vi "CloseUDP Connection.vi"(5 "UDP Network Connection Refnum":refnum<k16>) -> ()   [LabVIEW 2013]
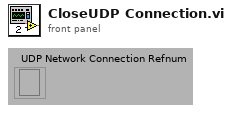
[diagram p1: front panel]
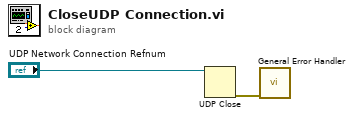
[diagram p0: block diagram]
diagram:
  n1 = UDP Close(connection ID="UDP Network Connection Refnum") -> (error out=w2:errorcluster)  [unwired: 1 in, 1 out]
  n2 = call <vilib>:"General Error Handler.vi"("error in (no error)"=w2) -> ()  [unwired: 1 in, 14 out]
